vi "NewVSS_GoTo.vi"(7 "Position":dbl[](array[numeric]), 8 "Path  Smooth":dbl[][](array[numeric]), 9 "orientation":dbl, 10 "V_tan":dbl, 11 "V_xy":dbl[](array[numeric])) -> (3 "Output Velocity":dbl[](array[numeric]) format="%.2f")   [LabVIEW 2018]
uses:
  <vilib>/Analysis/coordinate.llb/2D Cartesian Coordinate Rotation (Scalar).vi
  <vilib>/Analysis/NI_AALPro.lvlib
panel:
  in  "Limits":cluster{"output high":dbl, "output low":dbl}
  in  "PID gains in":T1={"proportional gain (Kc)"=2.0, "integral time (Ti, min)"=0.0, "derivative time (Td, min)"=10.0}
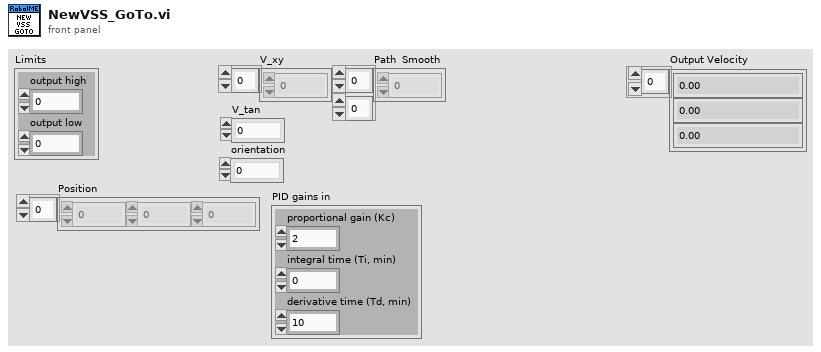
[diagram p1: front panel]
types:
  T1 = cluster{"proportional gain (Kc)":dbl, "integral time (Ti, min)":dbl, "derivative time (Td, min)":dbl}
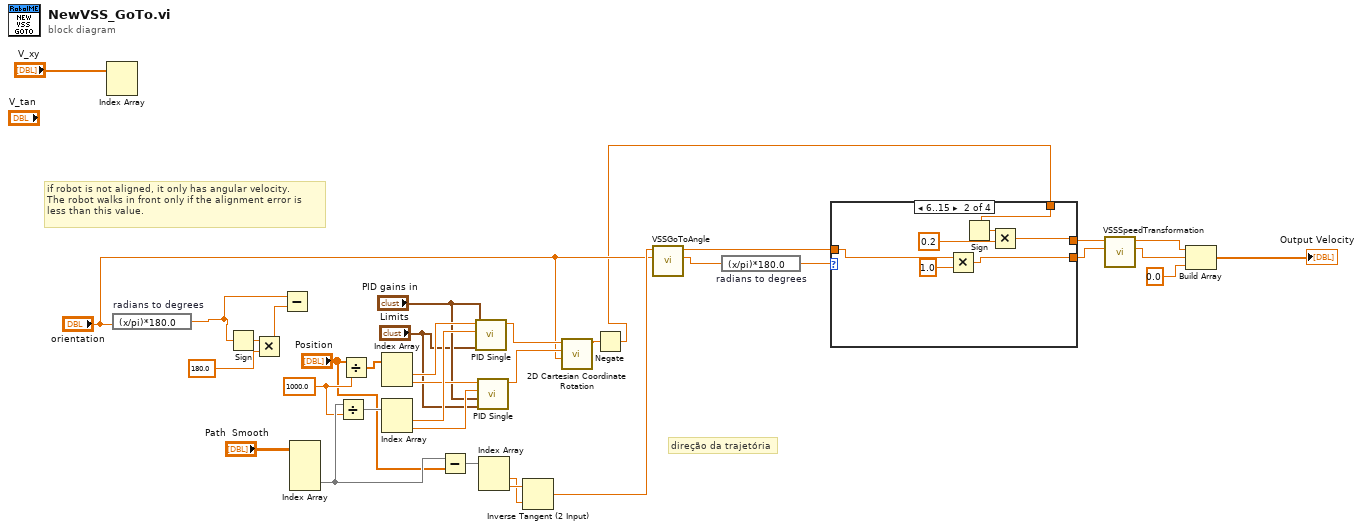
[diagram p0: block diagram]
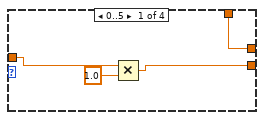
[diagram p2: hidden frame]
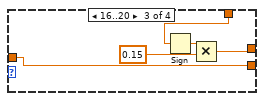
[diagram p3: hidden frame]
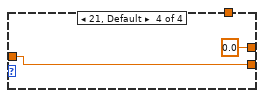
[diagram p4: hidden frame]
diagram:
  w5 = 1000.0
  # "direção da trajetória"
  # "if robot is not aligned, it only has angular velocity.\nThe robot walks in front only if the alignment error is\nless than this value."
  n1 = Index Array(array="V_xy") -> ()  [unwired: 2 in, 2 out]
  n2 = expression code="(x/pi)*180.0" "radians to degrees"("orientation") -> (w27:dbl)
  n3 = Sign(1:w27) -> (0:w29:dbl)
  n4 = Multiply(x=w29, y=180.0) -> (x*y=w28:dbl)
  n5 = Subtract(x=w27, y=w28) -> ()  [unwired: 1 out]
  n6 = Index Array(array="Path  Smooth") -> (element #2=w6:dbl[])  [unwired: 4 in, 1 out]
  n7 = Divide(x=w6, y=w5) -> (x/y=w7:dbl[])
  n8 = Divide(x="Position", y=w5) -> (x/y=w8:dbl[])
  n9 = Index Array(array=w8) -> (element #1=w18:dbl, element #2=w16:dbl)  [unwired: 2 in]
  n10 = Index Array(array=w7) -> (element #1=w17:dbl, element #2=w15:dbl)  [unwired: 2 in]
  n11 = Subtract(x=w6, y="Position") -> (x-y=w22:dbl[])
  n12 = call "PID Single.vi"("Limits"="Limits", "PID gains in"="PID gains in", "Variable"=w17, "Setpoint"=w18) -> ("Out"=w12:dbl)  [unwired: 7 in]
  n13 = call "PID Single.vi"("Limits"="Limits", "PID gains in"="PID gains in", "Variable"=w15, "Setpoint"=w16) -> ("Out"=w11:dbl)  [unwired: 7 in]
  n14 = Index Array(array=w22) -> (element #1=w20:dbl, element #2=w21:dbl)  [unwired: 2 in]
  n15 = Inverse Tangent (2 Input)(1:w20, 2:w21) -> (0:w19:dbl)
  n16 = call-poly <vilib>:"2D Cartesian Coordinate Rotation.vi"("theta"="orientation", "y"=w11, "x"=w12) -> ("x out"=w9:dbl)  [unwired: 6 in, 2 out]
  n17 = Negate(x=w9) -> (-x=w4:dbl)
  n18 = call "VSSGoToAngle.vi"("orientation"="orientation", "dest_orientation"=w19) -> ("AngleError"=w26:dbl, "v_ang"=w3:dbl)  [unwired: 7 in, 1 out]
  n19 = expression code="(x/pi)*180.0" "radians to degrees"(w26) -> (w25:dbl)
  n20 = case shown="6..15" w25 {
    tunnel: [w37 w41 w51 w52] -> w24
    tunnel: w3 -> [w38 w42 w51 w52]
    tunnel: w4 -> [w39 w46 w48 _]
    tunnel: [w39 w44 w47 0.0] -> w2
    frame 0..5 {
      n21 = Multiply(x=w38, y=1.0) -> (x*y=w37:dbl)
    }
    frame 6..15 {
      n22 = Multiply(x=w42, y=1.0) -> (x*y=w41:dbl)
      n23 = Sign(1:w46) -> (0:w45:dbl)
      n24 = Multiply(x=w45, y=0.2) -> (x*y=w44:dbl)
    }
    frame 16..20 {
      n25 = Sign(1:w48) -> (0:w50:dbl)
      n26 = Multiply(x=w50, y=0.15) -> (x*y=w47:dbl)
    }
    frame 21, Default {
    }
  }
  n27 = call "VSSSpeedTransformation.vi"("V_ang in"=w24, "V_tang in"=w2) -> ("V_rigth"=w31:dbl, "V_left"=w32:dbl)  [unwired: 8 in]
  n28 = Build Array(w32, w31, 0.0 ("element")) -> (→"Output Velocity":dbl[])
